vi "Show With Fade In.vi"(8 "error in (no error)":errorcluster, 9 "Target Transparency (0)":u8, 10 "Fade time (800ms)":i32=800, 11 "Flex UI (Actor) in":refnum<class "Flex UI (Actor).lvclass">) -> (0 "error out":errorcluster, 3 "Flex UI (Actor) out":refnum<class "Flex UI (Actor).lvclass">)   [LabVIEW 2016, in "Flex UI (Parent Actor).lvlib" / "Flex UI (Actor).lvclass"]
uses:
  Flex UI (Actor).lvclass
  <vilib>/East West Architects/Flex UI/Flex UI (Parent)/Flex UI.lvclass
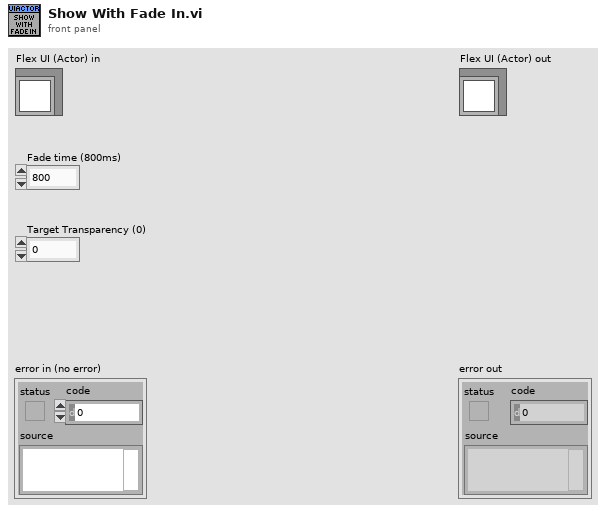
[diagram p1: front panel]
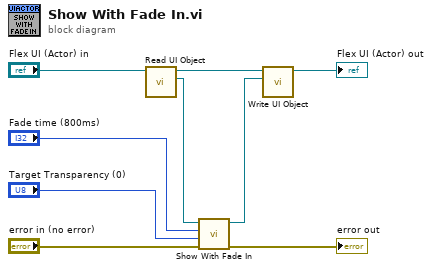
[diagram p0: block diagram]
diagram:
  n1 = call-dynamic "Read UI Object.vi"("Flex UI (Actor) in"="Flex UI (Actor) in") -> ("Flex UI Object"=w4:refnum<class "Flex UI.lvclass">, "Flex UI (Actor) out"=w5:refnum<class "Flex UI (Actor).lvclass">)  [unwired: 8 in, 1 out]
  n2 = call-dynamic "Show With Fade In.vi"("error in (no error)"="error in (no error)", "Target Transparency (100)"="Target Transparency (0)", "Fade time (800ms)"="Fade time (800ms)", "Flex UI in"=w4) -> ("error out"=→"error out":errorcluster, "Flex UI out"=w3:refnum<class "Flex UI.lvclass">)  [unwired: 6 in]
  n3 = call-dynamic "Write UI Object.vi"("Flex UI in"=w3, "Flex UI (Actor) in"=w5) -> ("Flex UI (Actor) out"=→"Flex UI (Actor) out":refnum<class "Flex UI (Actor).lvclass">)  [unwired: 8 in, 1 out]
